vi "OAT Track Orders in Resampled Signal (Multi Channels).vi"(0 "resample signals":cluster{"r0":dbl, "dr":dbl, "Y":dbl[]}[](array[cluster]) {"r0" format="%.2p"; "dr" format="%.2p"; "Y" format="%.2f"}, 1 "orders (1.0)":dbl[](array[numeric])=[1.0] format="%.2f", 2 "X axis selection":u16(ring)=2 items=["Time", "Revolution", "RPM"], 3 "reset? (True)":bool=TRUE, 5 "channel info":T2[](array[typedef]) {"pregain" format="%.2f"; "weighting filter" items=["Linear", "A-weighting", "B-weighting", "C-weighting", "ITU-R 468-4", "Dolby", "CCITT", "C-message", "Wb", "Wc", "Wd", "We", "Wf", "Wh", "Wj", "Wk", "Wm", "AES17 20 kHz lowpass", "AES17 40 kHz lowpass", "AES17 20 kHz highpass", "AES17 40 kHz highpass"]; "dB reference" format="%^.1e"; "engineering units" items=["custom..."=0, "V"=1, "A"=21, "C"=30, "pC"=31, "s"=32, "-"=29, "Pa"=2, "N"=20, "g"=3, "m/s^2"=4, "m/s"=5, "m"=6, "mm/s"=12, "mm"=13, "micron/s"=14, "micron"=15, "in/s^2"=7, "in/s"=8, "in"=9, "mil/s"=10, "mil"=11, "rad/s^2"=16, "rad/s"=17, "rad"=18, "deg/s^2"=26, "deg/s"=27, "deg"=28, "RPM"=22, "cycle/s^2"=23, "Hz"=24, "cycle"=25, "strain"=19]; "sensor sensitivity" format="%#_5f"}, 7 "time instant":dbl[](array[numeric]) format="%.2f", 11 "error in (no error)":errorcluster, 12 "bandwidth [order]":dbl format="%.2f", 13 "phase setting":T5) -> (4 "magnitudes (RMS)":cluster{"X":dbl[], "Y":dbl[]}[][](array[cluster]) {"Y" format="%.2f"; "X" format="%.2f"}, 6 "phase lags":cluster{"X":dbl[], "Y":dbl[]}[][](array[cluster]) {"Y" format="%.2f"; "X" format="%.2f"}, 8 "samples/rev":dbl format="%.2f", 10 "unit labels":T1(array[cluster]), 15 "error out":errorcluster)   [LabVIEW 2017]
doc: "Computes magnitudes and phases for designated orders from <B>resampled signal</B> of multiple channels."
uses:
  <vilib>/addons/_NISVFA/_Shared subVIs/Controls/svc_Channel Info.ctl
  <vilib>/addons/_NISVFA/_Shared subVIs/Controls/svc_Engineering Units Text Ring.ctl
  <vilib>/addons/_NISVFA/_Shared subVIs/Controls/svc_Weighting Filter Text Ring.ctl
  <vilib>/addons/Sound and Vibration/Order Analysis/Resample Order Tracking/SubVIs/OAT Order Magnitude and Phase Plot(XY) (Multi Channels).vi
  <vilib>/addons/Sound and Vibration/Order Analysis/Resample Order Tracking/SubVIs/OAT Demodulate Multiple Orders (Multi Channels).vi
  <vilib>/addons/Sound and Vibration/Order Analysis/Resample Order Tracking/SubVIs/OAT Verify Resampled Signal (Multi Channels).vi
  <vilib>/addons/Sound and Vibration/Order Analysis/Resample Order Tracking/SoundVib_Resampling.lvlib
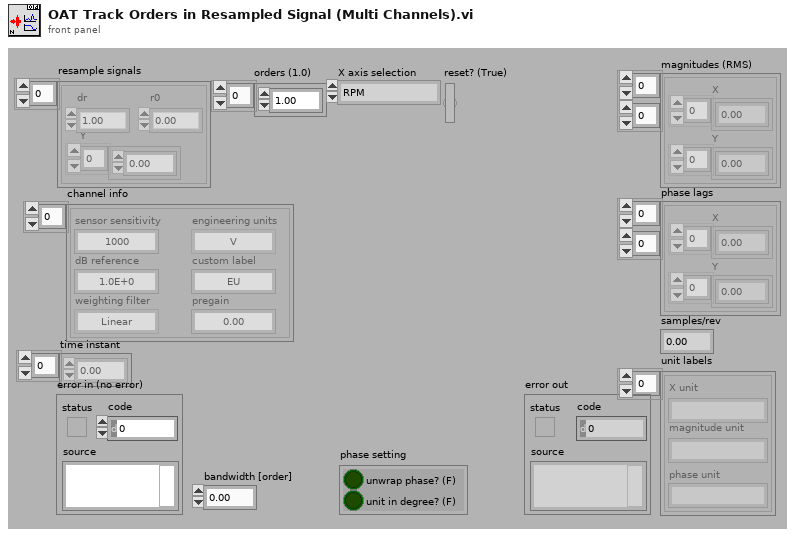
[diagram p1: front panel]
types:
  T1 = cluster{"X unit":string, "magnitude unit":string, "phase unit":string}[]
  T2 = typedef "svc_Channel Info.ctl" = cluster{"sensor sensitivity":dbl, "engineering units":T3, "dB reference":dbl, "custom label":string, "weighting filter":T4, "pregain":dbl}
  T3 = typedef "svc_Engineering Units Text Ring.ctl" = u16
  T4 = typedef "svc_Weighting Filter Text Ring.ctl" = u16
  T5 = cluster{"unwrap phase? (F)":bool, "unit in degree? (F)":bool}
  T6 = cluster{"bandwidth [order]":dbl, "stop band attenuation":u16}
  T7 = cluster{"X unit":string, "unit label":string, "unit label":string}[]
  T8 = typedef "SoundVib_TachProcess.lvlib/speed profile.ctl" = cluster{"time [s]":dbl[], "speed [RPM]":dbl[]}
  T9 = cluster{"X unit":string, "unit label":string, "unit label":string}
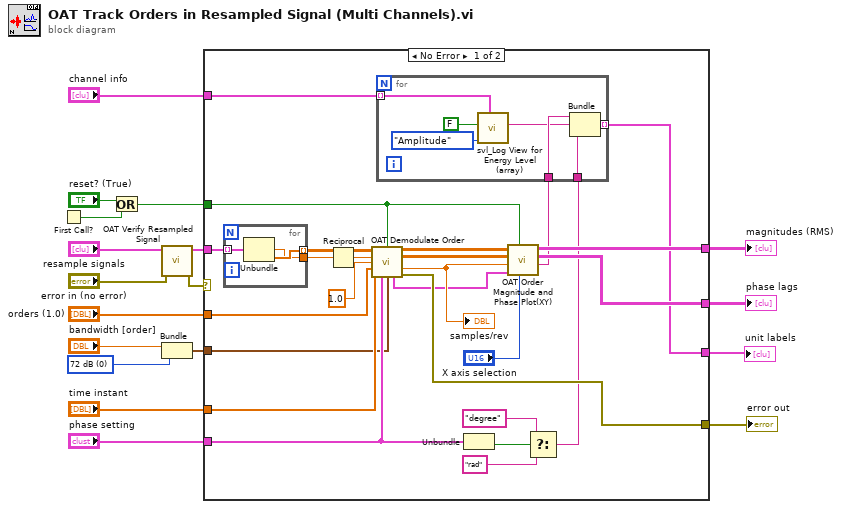
[diagram p0: block diagram]
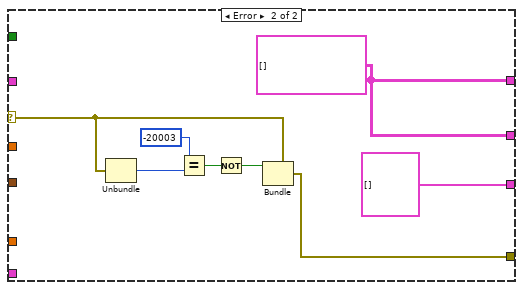
[diagram p2: hidden frame]
diagram:
  w2 = u16 0 items=["72 dB", "96 dB", "120 dB"] ("stop band attenuation")
  n1 = First Call?() -> (First Call?: T/F=w7:bool)
  n2 = Or(x="reset? (True)", y=w7) -> (x .or. y?=w6:bool)
  n3 = call-poly <vilib>:"OAT Verify Resampled Signal.vi"("error in (no error)"="error in (no error)", "resampled signal"="resample signals") -> ("error out"=w11:errorcluster, "resampled signal out"=w12:cluster{"r0":dbl, "dr":dbl, "Y":dbl[]}[])  [unwired: 7 in, 1 out]
  n4 = Bundle("bandwidth [order]"="bandwidth [order]", "stop band attenuation"=w2) -> (w1:T6)  [unwired: 1 in]
  n5 = case shown="No Error" w11 {
    selector: w11 -> [_ w57]
    tunnel: "orders (1.0)" -> [w38 _]
    tunnel: [w27 T7 []] -> w4
    tunnel: "time instant" -> [w43 _]
    tunnel: "phase setting" -> [w39 _]
    tunnel: [w42 w61] -> w15
    tunnel: [w41 w61] -> w14
    tunnel: w6 -> [w40 _]
    tunnel: w12 -> [w21 _]
    tunnel: [w37 w54] -> w10
    tunnel: "channel info" -> [w22 _]
    tunnel: w1 -> [w24 _]
    frame No Error {
      n6 = for {
        tunnel: w21 -> [w46] mode=indexing
        tunnel: [w45] -> w20 mode=indexing
        tunnel: [w44] -> w19
        n7 = Unbundle(w46) -> ("dr"=w44:dbl, "Y"=w45:dbl[])  [unwired: 1 out]
      }
      n8 = Reciprocal(x=w19) -> (1/x=w31:dbl)
      n9 = call-poly <vilib>:"OAT Demodulate Order.vi"("Y"=w20, "reset? (True)"=w40, "samples/rev"=w31, "samples/rev wanted"=1.0 ("x"), "orders (1.0)"=w38, "time stamps in"=w43, "phase setting"=w39, "order info"=w24) -> ("magnitudes (RMS)"=w26:dbl[][][], "phase lag"=w25:dbl[][][], "samples/rev"=w32:dbl, "speed profile"=w30:T8, "error out"=w37:errorcluster)  [unwired: 3 in]
      "samples/rev" <- w32
      n10 = Unbundle(w39) -> ("unit in degree? (F)"=w36:bool)  [unwired: 1 out]
      n11 = call-poly <vilib>:"OAT Order Magnitude and Phase Plot(XY).vi"("X axis selection"="X axis selection", "reset? (True)"=w40, "speed profile"=w30, "samples/rev"=w32, "phase lag  (even angular)"=w25, "magnitudes (even angular)"=w26) -> ("X unit"=w29:string, "phase lag"=w42:cluster{"X":dbl[], "Y":dbl[]}[][], "magnitudes"=w41:cluster{"X":dbl[], "Y":dbl[]}[][])  [unwired: 3 in]
      n12 = Select(t="degree" ("unit label"), s=w36, f="rad" ("unit label")) -> (s? t:f=w28:string)
      n13 = for {
        tunnel: w29 -> [w53]
        tunnel: w28 -> [w52]
        tunnel: [w51] -> w27 mode=indexing
        tunnel: w22 -> [w47] mode=indexing
        n14 = call <vilib>:"svl_Log View for Energy Level (array).vi"("channel info"=w47, "view mode"=enum16{"Power", "Amplitude"}."Amplitude", "dB On (T)"=FALSE) -> ("unit label"=w50:string)  [unwired: 6 in, 2 out]
        n15 = Bundle("X unit"=w53, "unit label"=w50, "unit label"=w52) -> (w51:T9)  [unwired: 1 in]
      }
    }
    frame Error {
      w61 = cluster{"X":dbl[], "Y":dbl[]}[][] [] ("magnitudes")
      n16 = Unbundle(w57) -> ("code"=w59:i32)  [unwired: 2 out]
      n17 = Equal?(x=-20003 ("t"), y=w59) -> (x = y?=w56:bool)
      n18 = Not(x=w56) -> (.not. x?=w55:bool)
      n19 = Bundle(cluster=w57, "status"=w55) -> (w54:errorcluster)  [unwired: 2 in]
    }
  }
  "magnitudes (RMS)" <- w14
  "phase lags" <- w15
  "error out" <- w10
  "unit labels" <- w4
